vi "fit_transform.vi"(8 "error in (no error)":errorcluster caption="entrée d'erreur (pas d'erreur)", 11 "EnsembleBlender.lvclass 2":refnum<class "EnsembleBlender.lvclass">) -> (0 "error out":errorcluster caption="sortie d'erreur", 2 "X_new":dbl[][](array[numeric]), 3 "EnsembleBlender.lvclass":refnum<class "EnsembleBlender.lvclass">)   [LabVIEW 2020, in "EnsembleBlender.lvclass"]
doc: "Fit to data, then transform it.\n\n Fits transformer to `X` and `y` with optional parameters `fit_params`\n and returns a transformed version of `X`."
uses:
  EnsembleBlender.lvclass
  C:/Users/cipop/TDF Dropbox/2_Technologies de France/1 - Services et Etudes/PLAIY/2 - DEV/PLAIYLAB/code/Python/Python.lvclass
  C:/Users/cipop/TDF Dropbox/2_Technologies de France/1 - Services et Etudes/PLAIY/2 - DEV/PLAIYLAB/code/Model/Model.lvclass
  C:/Users/cipop/TDF Dropbox/2_Technologies de France/1 - Services et Etudes/PLAIY/2 - DEV/PLAIYLAB/code/Model/Supervised/Ensemble/Ensemble.lvclass
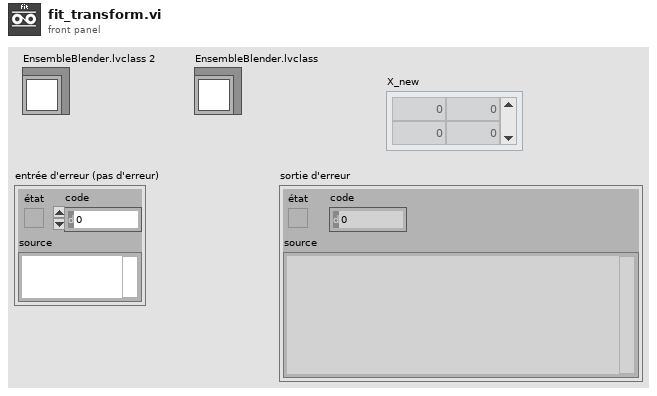
[diagram p1: front panel]
types:
  T1 = typedef "data.ctl" = cluster{"name":string, "X":dbl[][]}
  T2 = typedef "ensemble_data.ctl" = cluster{"y":dbl[], "sample_weight":dbl[]}
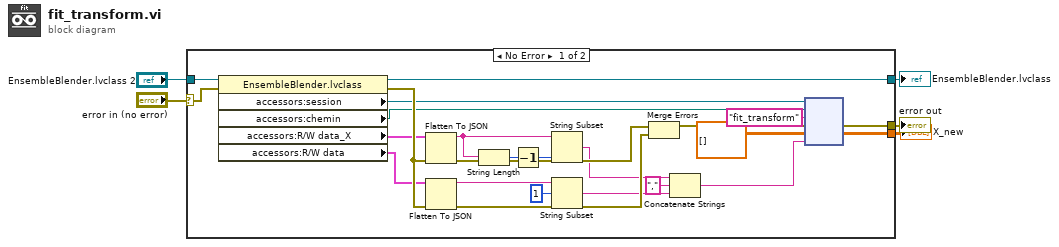
[diagram p0: block diagram]
diagram:
  n1 = case shown="No Error" "error in (no error)" {
    selector: "error in (no error)" -> [w27 w31]
    tunnel: [w28 w31] -> w4
    tunnel: [w10 w30] -> w2
    tunnel: "EnsembleBlender.lvclass 2" -> [w9 w30]
    tunnel: [w7 _] -> w1
    frame No Error {
      n2 = property class="EnsembleBlender.lvclass"(reference=w9, error in=w27) -> (reference out=w10:refnum<class "EnsembleBlender.lvclass">, error out=w23:errorcluster, "accessors:session"=w13:refnum<k35>, "accessors:chemin"=w12:path, "accessors:R/W data_X"=w14:T1, "accessors:R/W data"=w6:T2)
      n3 = Flatten To JSON(anything=w14, error in (no error)=w23) -> (JSON string=w24:string, 11:w19:errorcluster)  [unwired: 1 in]
      n4 = Flatten To JSON(anything=w6, error in (no error)=w23) -> (JSON string=w21:string, 11:w20:errorcluster)  [unwired: 1 in]
      n5 = String Length(string=w24) -> (length=w26:i32)
      n6 = Decrement(x=w26) -> (x-1=w25:i32)
      n7 = String Subset(string=w24, length (rest)=w25) -> (substring=w17:string)  [unwired: 1 in]
      n8 = String Subset(string=w21, offset (0)=1) -> (substring=w16:string)  [unwired: 1 in]
      n9 = Merge Errors(w19, w20) -> (w11:errorcluster)
      n10 = Concatenate Strings(w17, "," ("string"), w16) -> (w15:string)
      n11 = node(w13, w12, "fit_transform" ("nom de la fonction"), w11, dbl[][] [], w15) -> (w28:errorcluster, w7:dbl[][])  [unwired: 1 in, 3 out]
    }
    frame Error {
    }
  }
  "error out" <- w4
  "EnsembleBlender.lvclass" <- w2
  "X_new" <- w1
